vi "CapacitanceNavigation.vi"() -> ()   [LabVIEW 2010]
uses:
  <userlib>/Nanonis Prog Interface V5/Nanonis Prog Interface.lvlib
panel:
  in  "pause":bool
  in  "Delete First Entry":bool
  in  "Time between averages (ms)":u32
  out "Avg index":i32
  in  "Averages":i32
  in  "milliseconds to wait":u32
  in  "stop":bool
  in  "?":bool
  in  "Max Steps":u16=500
  in  "Direction":enum16{"X +", "X -", "Y +", "Y -", "Z +", "Z -"}(ring)
  out "Delta":cluster{"index":i32, sgl}[](graph)
  in  "Number of Steps":u16=50
  out "Capacitance":cluster{"index":i32, sgl}[](graph)
  in  "Frequency (Hz)":sgl=261.0
  in  "Amplitude (V)":sgl=350.0
  # "Max Steps On"
  # "Max Steps Off"
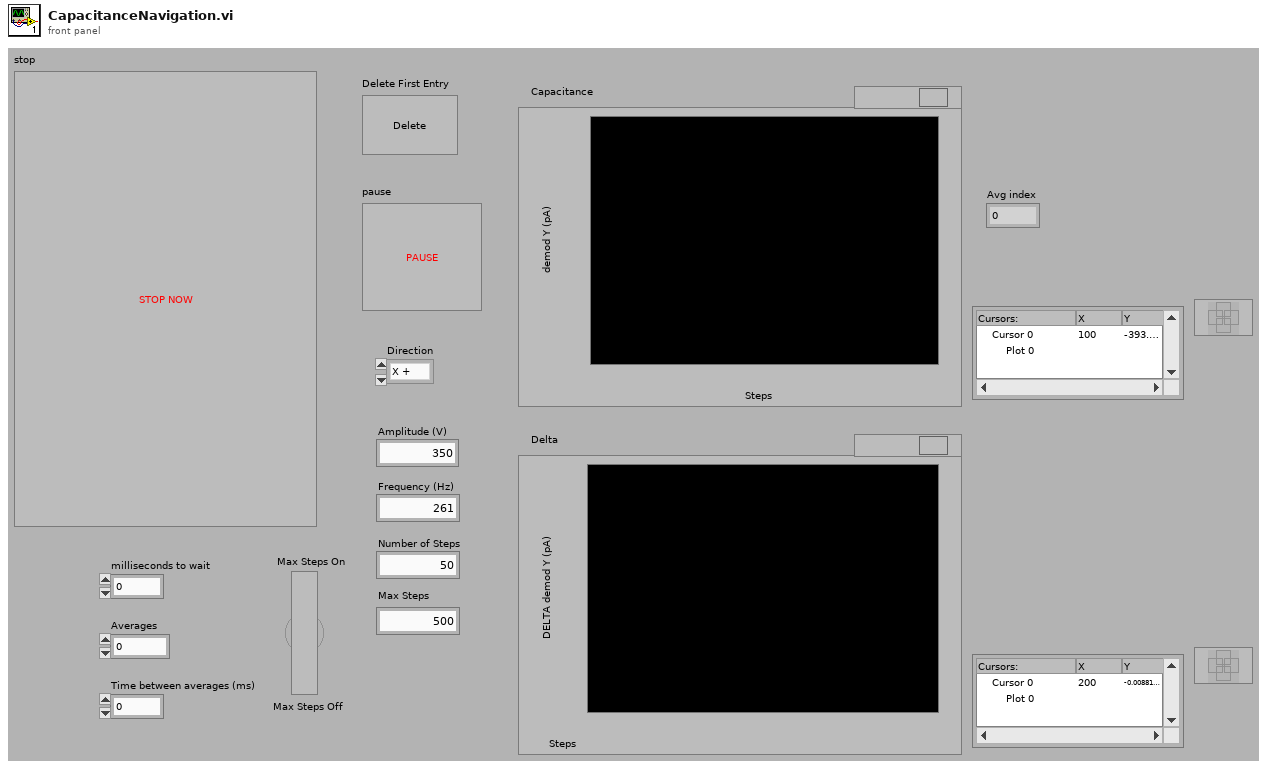
[diagram p1: front panel]
types:
  T1 = enum8{"Group 1", "Group 2", "Group 3", "Group 4", "Group 5", "Group 6"}
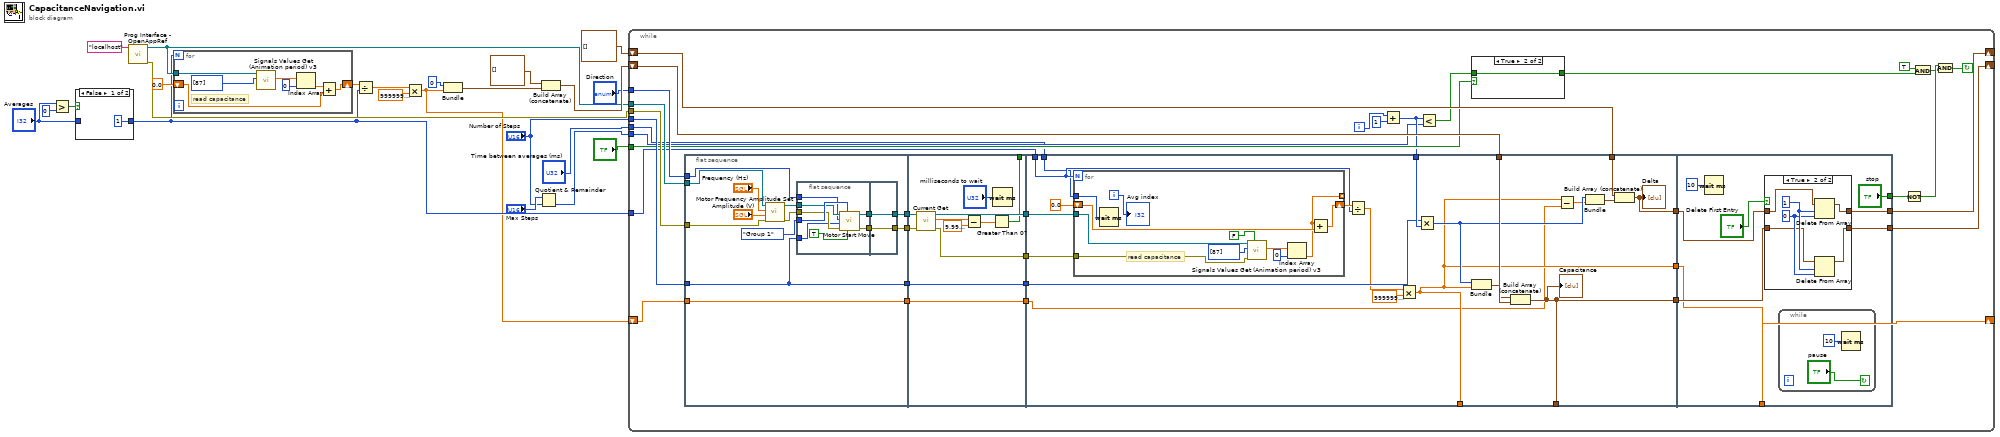
[diagram p0: block diagram]
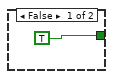
[diagram p3: hidden frame]
diagram:
  n1 = Greater?(x="Averages", y=0) -> (0:w8:bool)
  n2 = case shown="False" w8 {
    tunnel: "Averages" -> [_ w25]
    tunnel: [1 ("Averages") w25] -> w3
    frame False {
    }
    frame True {
    }
  }
  n3 = call <userlib>:"Prog Interface - OpenAppRef.vi"("Machine name (local machine IP)"="localhost" ("machine name (localhost)")) -> ("Error out"=w17:errorcluster, "Application reference"=w16:refnum<vi>)  [unwired: 5 in]
  n4 = for {
    N: w3 -> [_]
    tunnel: w16 -> [w29]
    shift-right: [w26] -> w4
    shift-left: sgl 0.0 ("Internal Ch Value") -> [w28]
    # "read capacitance"
    n5 = call <userlib>:"Signals Values Get (Animation period) v3.vi"("Signals indexes (0-127)"=i8[] [87], "Application ref in"=w29) -> ("Signals Values"=w30:sgl[])  [unwired: 6 in, 2 out]
    n6 = Index Array(array=w30, index=0) -> (element=w27:sgl)
    n7 = Add(x=w27, y=w28) -> (x+y=w26:sgl)
  }
  n8 = Divide(x=w4, y=w3) -> (x/y=w2:sgl)
  n9 = Multiply(x=w2, y=sgl 1000000000000.0) -> (x*y=w1:sgl)
  n10 = Bundle("index"=0, w1) -> (w20:cluster{"index":i32, sgl})  [unwired: 1 in]
  n11 = Quotient & Remainder(x="Max Steps", y="Number of Steps") -> (floor(x/y)=w11:u16)  [unwired: 1 out]
  n12 = Build Array (concatenate)(cluster{i32, sgl}[] [], w20) -> (w19:cluster{"index":i32, sgl}[])
  n13 = while {
    shift-right: [w38] -> _
    shift-left: w19 -> [w65]
    tunnel: w16 -> [w63]
    tunnel: w17 -> [w62]
    shift-right: [w56] -> _
    shift-left: cluster{i32, sgl}[] [] -> [w55]
    tunnel: "Direction" -> [w54]
    tunnel: "Number of Steps" -> [w53]
    tunnel: w11 -> [w46]
    tunnel: "?" -> [w52]
    tunnel: w3 -> [w41]
    tunnel: "Time between averages (ms)" -> [w40]
    shift-right: [w36] -> _
    shift-left: w1 -> [w35]
    i -> [w49]
    stop <- w43 continue-if-true
    n14 = flat-sequence {
      tunnel: [w72] -> w67
      tunnel: w63 -> [w75]
      tunnel: w62 -> [w78]
      tunnel: [w77] -> w61
      tunnel: [w76] -> w60
      tunnel: w54 -> [w71]
      tunnel: w53 -> [w72]
      tunnel: w35 -> [w70]
      tunnel: [w70] -> w34
      tunnel: w67 -> [w104]
      tunnel: [w104] -> w66
      tunnel: w61 -> [w103]
      tunnel: w60 -> [w102]
      tunnel: [w101] -> w59
      tunnel: [w100] -> w58
      tunnel: [w97] -> _
      tunnel: w34 -> [w94]
      tunnel: [w94] -> w33
      tunnel: [w107] -> _
      tunnel: w47 -> [w123]
      tunnel: w66 -> [w120]
      tunnel: w65 -> [w121]
      tunnel: [w106] -> _
      tunnel: w59 -> [w119]
      tunnel: w58 -> [w118]
      tunnel: [w114] -> w57
      tunnel: w55 -> [w115]
      tunnel: w41 -> [w109]
      tunnel: w40 -> [w108]
      tunnel: [w107] -> w39
      tunnel: [w106] -> w37
      tunnel: w33 -> [w105]
      tunnel: w57 -> [w140]
      tunnel: [w139] -> w56
      tunnel: ["stop"] -> w42
      tunnel: [w137] -> w38
      tunnel: w39 -> [w138]
      tunnel: w37 -> [w136]
      tunnel: [w136] -> w36
      frame #0 {
        n15 = call <userlib>:"Motor Frequency Amplitude Set.vi"("Error in (no error)"=w78, "Amplitude (V) (NaN=no change)"="Amplitude (V)", "Frequency (Hz) (NaN=no change)"="Frequency (Hz)", "Application ref in"=w75) -> ("Error out"=w79:errorcluster, "Application ref out"=w80:refnum<vi>)  [unwired: 6 in]
        n16 = flat-sequence {
          tunnel: T1."Group 1" ("Group") -> [w90]
          tunnel: w80 -> [w89]
          tunnel: w79 -> [w88]
          tunnel: w72 -> [w87]
          tunnel: [w86] -> w74
          tunnel: [w85] -> w73
          tunnel: w71 -> [w84]
          tunnel: [w92] -> w76
          tunnel: [w93] -> w77
          tunnel: w74 -> [w93]
          tunnel: w73 -> [w92]
          frame #0 {
            n17 = call <userlib>:"Motor Start Move.vi"("Wait until finished? (F)"=TRUE, "Group"=w90, "Error in (no error)"=w88, "Number of steps"=w87, "Direction"=w84, "Application ref in"=w89) -> ("Error out"=w85:errorcluster, "Application ref out"=w86:refnum<vi>)  [unwired: 3 in]
          }
          frame #1 {
          }
        }
      }
      frame #1 {
        n18 = call <userlib>:"Current Get.vi"("Error in (no error)"=w102, "Application ref in"=w103) -> ("Error out"=w101:errorcluster, "Current (A)"=w99:sgl, "Application ref out"=w100:refnum<vi>)  [unwired: 5 in]
        n19 = Subtract(x=w99, y=sgl 1e-09) -> (x-y=w98:sgl)
        n20 = Greater Than 0?(x=w98) -> (x > 0?=w97:bool)
        n21 = Wait (ms)(milliseconds to wait="milliseconds to wait") -> ()  [unwired: 1 out]
      }
      frame #2 {
        n22 = for {
          N: w109 -> [_]
          tunnel: w119 -> [w132]
          tunnel: w118 -> [w131]
          shift-right: [w129] -> w111
          shift-left: sgl 0.0 ("y") -> [w130]
          tunnel: w108 -> [w127]
          tunnel: [w125] -> _ mode=indexing
          i -> [w128]
          # "read capacitance"
          n23 = Wait (ms)(milliseconds to wait=w127) -> ()  [unwired: 1 out]
          n24 = call <userlib>:"Signals Values Get (Animation period) v3.vi"("Wait for newest data (F=False)"=FALSE, "error in (no error)"=w132, "Signals indexes (0-127)"=i8[] [87], "Application ref in"=w131) -> ("Signals Values"=w133:sgl[])  [unwired: 4 in, 2 out]
          n25 = Index Array(array=w133, index=0) -> (element=w125:sgl)
          n26 = Add(x=w125, y=w130) -> (x+y=w129:sgl)
          "Avg index" <- w128
        }
        n27 = Divide(x=w111, y=w109) -> (x/y=w110:sgl)
        n28 = Multiply(x=w110, y=sgl 1000000000000.0) -> (x*y=w106:sgl)
        n29 = Multiply(x=w120, y=w123) -> (x*y=w117:i32)
        n30 = Bundle(w117, w106) -> (w122:cluster{i32, sgl})  [unwired: 1 in]
        n31 = Build Array (concatenate)(w121, w122) -> (w107:cluster{"index":i32, sgl}[])
        "Capacitance" <- w107
        n32 = Subtract(x=w106, y=w105) -> (x-y=w113:sgl)
        n33 = Bundle(w117, w113) -> (w116:cluster{i32, sgl})  [unwired: 1 in]
        n34 = Build Array (concatenate)(w115, w116) -> (w114:cluster{i32, sgl}[])
        "Delta" <- w114
      }
      frame #3 {
        n35 = Wait (ms)(milliseconds to wait=u32 10) -> ()  [unwired: 1 out]
        n36 = case shown="True" "Delete First Entry" {
          tunnel: w140 -> [w147 w151]
          tunnel: [w147 w150] -> w139
          tunnel: w138 -> [w146 w148]
          tunnel: [w146 w149] -> w137
          frame False {
          }
          frame True {
            w153 = 1 ("length")
            w152 = 0 ("index")
            n37 = Delete From Array(array=w151, length=w153, index=w152) -> (array with subset deleted=w150:cluster{i32, sgl}[])  [unwired: 1 out]
            n38 = Delete From Array(array=w148, length=w153, index=w152) -> (array with subset deleted=w149:cluster{"index":i32, sgl}[])  [unwired: 1 out]
          }
        }
        n39 = while {
          stop <- "pause" continue-if-true
          n40 = Wait (ms)(milliseconds to wait=u32 10) -> ()  [unwired: 1 out]
        }
      }
    }
    n41 = Add(x=w49, y=u16 1) -> (x+y=w47:i32)
    n42 = Less?(x=w47, y=w46) -> (x < y?=w48:bool)
    n43 = case shown="True" w52 {
      tunnel: w48 -> [_ w69]
      tunnel: [TRUE w69] -> w50
      frame False {
      }
      frame True {
      }
    }
    n44 = Not(x=w42) -> (.not. x?=w45:bool)
    n45 = And(x=TRUE, y=w50) -> (x .and. y?=w44:bool)
    n46 = And(x=w45, y=w44) -> (x .and. y?=w43:bool)
  }
